vi "RedefineMasterIP.vi"() -> (1 "Abort?":bool)   [LabVIEW 2014]
doc: "Returns the current Master IP and port.\n\nUser has the option to change the address and/or port or make themselves the master"
uses:
  <userlib>/ROS for LabVIEW Software.lnk/ROS/Code/_ROSDefinition.vi
panel:
  in  "Cancel Button":bool
  in  "OK Button":bool
  in  "Address":string(combo)
  # "Please enter your Master IP address."
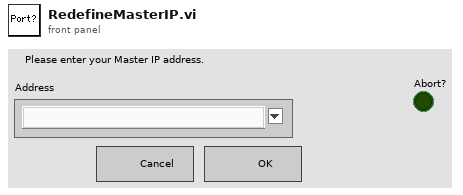
[diagram p1: front panel]
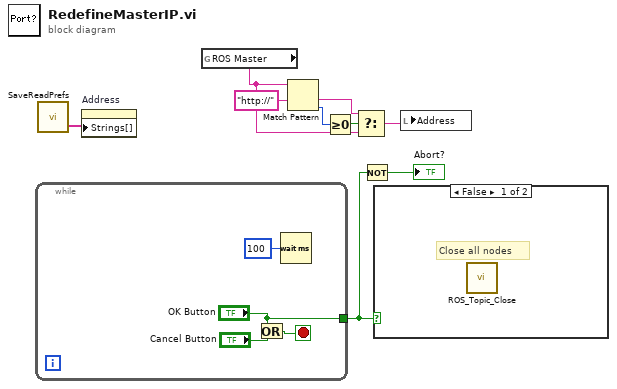
[diagram p0: block diagram]
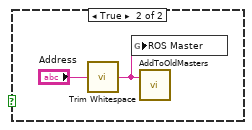
[diagram p2: hidden frame]
diagram:
  n1 = while {
    tunnel: ["OK Button"] -> w9
    stop <- w12 stop-if-true
    n2 = Or(x="OK Button", y="Cancel Button") -> (x .or. y?=w12:bool)
    n3 = Wait (ms)(milliseconds to wait=u32 100) -> ()  [unwired: 1 out]
  }
  n4 = call <userlib>:"SaveReadPrefs.vi"() -> ("Masters"=w2:string[])  [unwired: 3 in]
  n5 = property on="Address" class="CmbBox"("Strings[]"=w2) -> ()  [unwired: 2 in, 2 out]
  n6 = global read "_ROSDefinition.vi" "ROS Master"() -> (w3:string)
  n7 = Match Pattern(string=w3, regular expression="http://") -> (after substring=w4:string, offset past match=w6:i32)  [unwired: 1 in, 2 out]
  n8 = Greater Or Equal To 0?(x=w6) -> (x >= 0?=w5:bool)
  n9 = Select(t=w4, s=w5, f=w3) -> (s? t:f=w1:string)
  n10 = Not(x=w9) -> (.not. x?=→"Abort?":bool)
  n11 = case shown="False" w9 {
    frame False {
      # "Close all nodes"
      n12 = call <userlib>:"ROS_Topic_Close.vi"() -> ()  [unwired: 4 in, 1 out]
    }
    frame True {
      n13 = call <vilib>:"Trim Whitespace.vi"("string"="Address") -> ("trimmed string"=w14:string)  [unwired: 1 in]
      n14 = global write "_ROSDefinition.vi" "ROS Master"(w14) -> ()
      n15 = call <userlib>:"AddToOldMasters.vi"("Address"=w14) -> ()  [unwired: 3 in]
    }
  }
  n16 = local write "Address"(w1) -> ()
